vi "Format Part Caption Bold.vi"(0 "Bold Text":string, 1 "Caption Text \nIncluding Bold":string, 2 "Caption reference":refnum<vi>) -> ()   [LabVIEW 2025]
doc: "Author: Scott Hannahs <sth@magnet.fsu.edu>\n\nThis software is licensed for use under the “MIT License\"\nCopyright (c) 2025 Scott Hannahs, sth@sth@magnet.sthnet.net\n\nPermission is hereby granted, free of charge, to any person obtaining a copy of this software and associated documentation files (the \"Software\"), to deal in the Software without restriction, including without limitation the rights to use, copy, modify, merge, publish, distribute, sublicense, and/or sell copies of the Software, and to permit persons to whom the Software is furnished to do so, subject to the following conditions: The above copyright notice and this permission notice shall be included in all copies or substantial portions of the Software.\n\nTHE SOFTWARE IS PROVIDED \"AS IS\", WITHOUT WARRANTY OF ANY KIND, EXPRESS OR IMPLIED, INCLUDING BUT NOT LIMITED TO THE WARRANTIES OF MERCHANTABILITY, FITNESS FOR A PARTICULAR PURPOSE AND NONINFRINGEMENT. IN NO EVENT SHALL THE AUTHORS OR COPYRIGHT HOLDERS BE LIABLE FOR ANY CLAIM, DAMAGES OR OTHER LIABILITY, WHETHER IN AN ACTION OF CONTRACT, TORT OR OTHERWISE, ARISING FROM, OUT OF OR IN CONNECTION WITH THE SOFTWARE OR THE USE OR OTHER DEALINGS IN THE SOFTWARE."
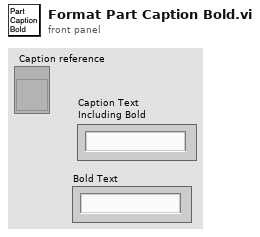
[diagram p1: front panel]
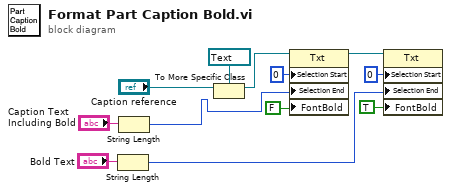
[diagram p0: block diagram]
diagram:
  n1 = String Length(string="Bold Text") -> (length=w1:i32)
  n2 = String Length(string="Caption Text \nIncluding Bold") -> (length=w2:i32)
  n3 = To More Specific Class(target class=refnum<vi> refnum ("String"), reference="Caption reference") -> (specific class reference=w10:refnum<vi>)  [unwired: 1 in, 1 out]
  n4 = property class="Txt"(reference=w10, "Selection Start"=u32 0 ("Selection:Start"), "Selection End"=w2, "FontBold"=FALSE ("Font:Bold")) -> (reference out=w7:refnum<vi>)  [unwired: 1 in, 1 out]
  n5 = property class="Txt"(reference=w7, "Selection Start"=u32 0 ("Selection:Start"), "Selection End"=w1, "FontBold"=TRUE) -> ()  [unwired: 1 in, 2 out]
